vi "JSONtext Pretty Print.vi"(11 "JSON":string) -> (2 "Value String":string, 3 "Boolean":bool)   [LabVIEW 2020]
uses:
  <vilib>/JDP Science/JSONtext/JSONtext.lvlib
panel:
  out "String":string
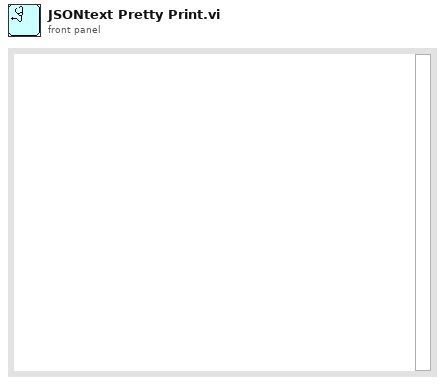
[diagram p1: front panel]
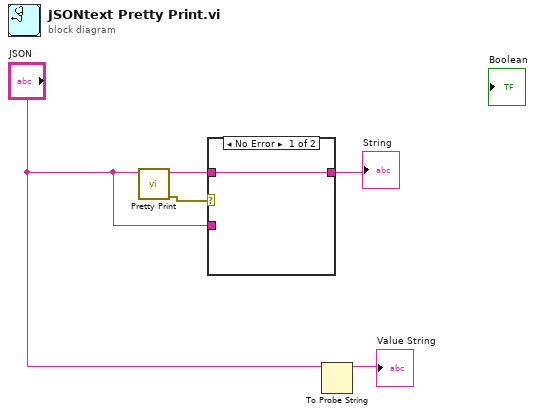
[diagram p0: block diagram]
diagram:
  n1 = call <vilib>:"Pretty Print.vi"("JSON"="JSON") -> ("error out"=w4:errorcluster, "<JSON>"=w3:string)  [unwired: 8 in, 1 out]
  n2 = case shown="No Error" w4 {
    tunnel: [w6 w7] -> w2
    tunnel: w3 -> [w6 _]
    tunnel: "JSON" -> [_ w7]
    frame No Error {
    }
    frame Error {
    }
  }
  "String" <- w2
  n3 = To Probe String(7:"JSON") -> (3:→"Value String":string)  [unwired: 2 in, 1 out]
